vi "Key_Display.vi"(0 "Data In":T6 caption="单捞磐 涝仿", 2 "Display State In":T4 caption="叼胶敲饭捞 惑怕 涝仿", 3 "Container State":T5 caption="牧抛捞呈 惑怕") -> (6 "Data Out":T6 caption="单捞磐 免仿", 7 "Display State Out":T4 caption="叼胶敲饭捞 惑怕 免仿", 8 "Action":T3 caption="累诀")   [LabVIEW 2012, in "Key_Xcontrol.xctl"]
uses:
  Key_Xcontrol.xctl
  Key_Data.ctl
  <vilib>/_xctls/Container State.ctl
  Key_State.ctl
  <vilib>/_xctls/Action.ctl
  <vilib>/_xctls/XControlSupport.lvlib
panel:
  in  "牧飘费侩":T1
  in  "牢叼霸捞磐侩":T2
  out "DISPLAY":T7
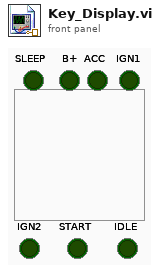
[diagram p1: front panel]
types:
  T1 = cluster{"SLEEP 2":bool, "B+ 2":bool, "ACC 2":bool, "IGN1 2":bool, "IGN2 2":bool, "START 2":bool, "IDLE 2":bool}
  T2 = cluster{"SLEEP":bool, "B+":bool, "ACC":bool, "IGN1":bool, "IGN2":bool, "START":bool, "IDLE":bool}
  T3 = typedef "XControlSupport.lvlib/Action.ctl" = cluster{"Data Changed?":bool, "State Changed?":bool, "Action Name":string}
  T4 = typedef "Key_Xcontrol.xctl/Key_State.ctl" = cluster{"Numeric":u8}
  T5 = typedef "XControlSupport.lvlib/Container State.ctl" = cluster{"Indicator?":bool, "Run Mode?":bool, " Refnum":refnum<vi>}
  T6 = typedef "Key_Xcontrol.xctl/Key_Data.ctl" = u8
  T7 = cluster{"Key In":bool, "acc":bool, "ign":bool, "start":bool}
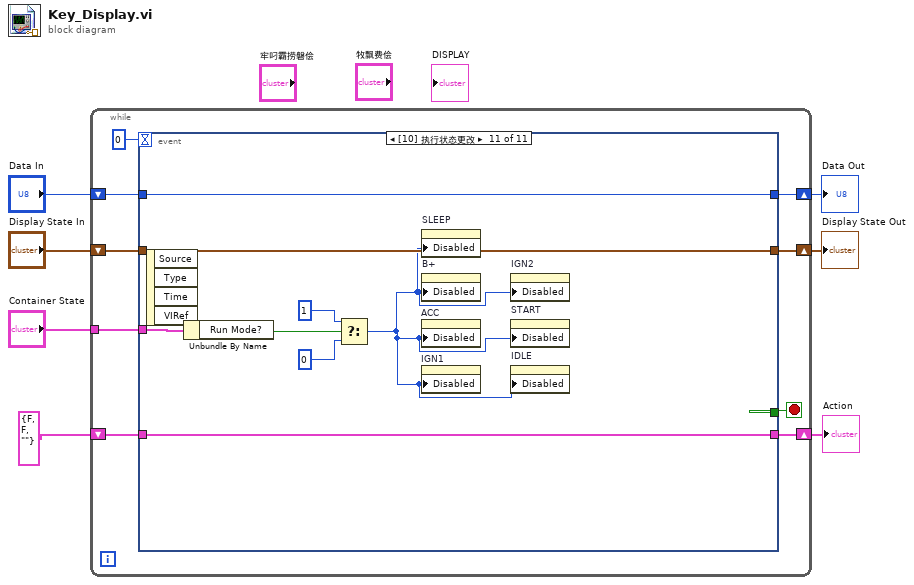
[diagram p0: block diagram]
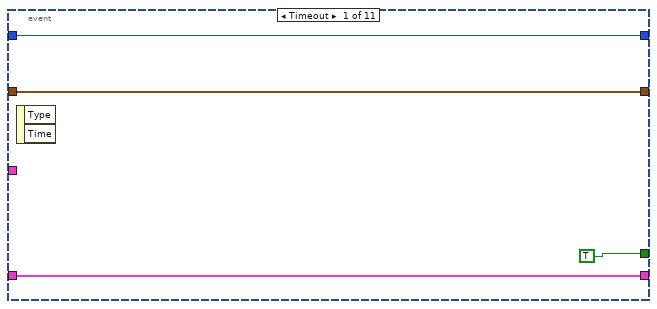
[diagram p2: hidden frame]
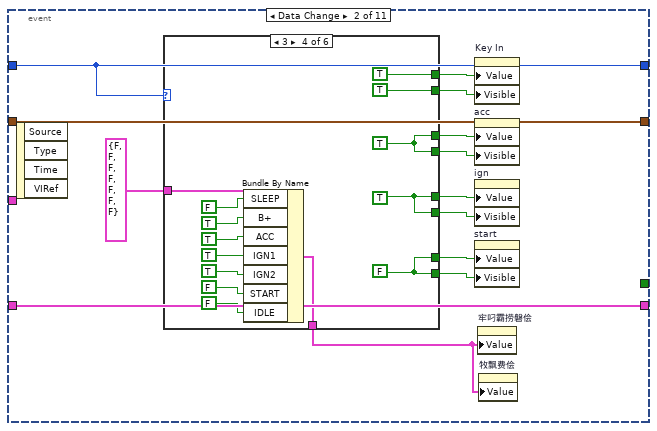
[diagram p3: hidden frame]
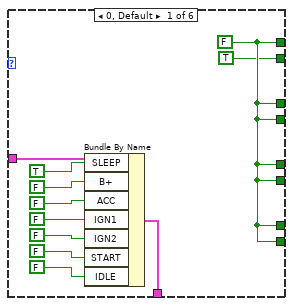
[diagram p4: hidden frame]
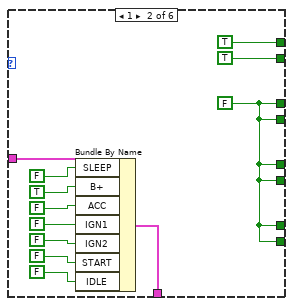
[diagram p5: hidden frame]
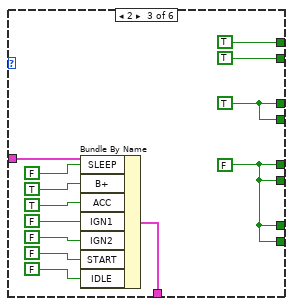
[diagram p6: hidden frame]
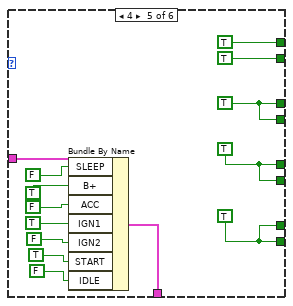
[diagram p7: hidden frame]
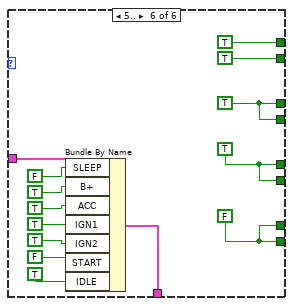
[diagram p8: hidden frame]
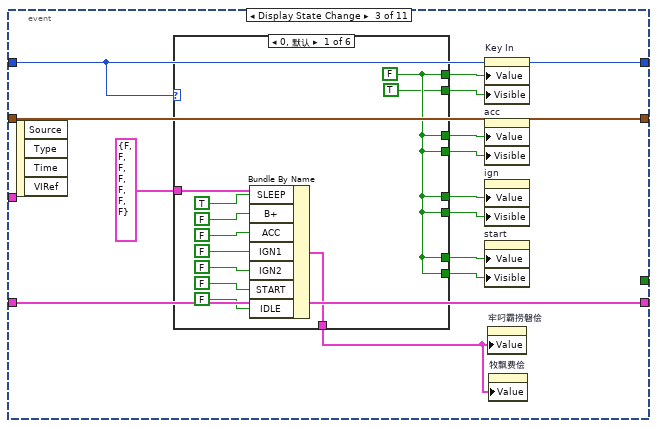
[diagram p9: hidden frame]
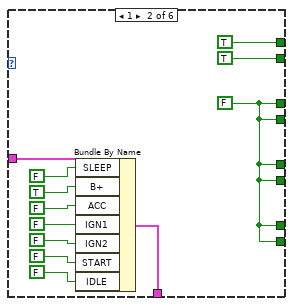
[diagram p10: hidden frame]
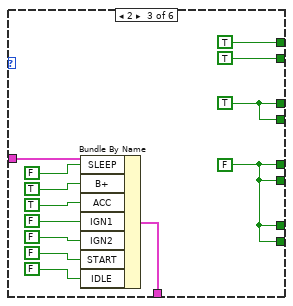
[diagram p11: hidden frame]
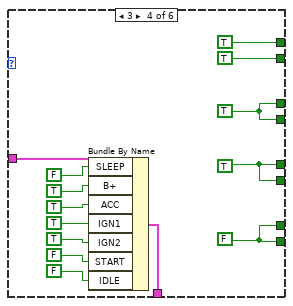
[diagram p12: hidden frame]
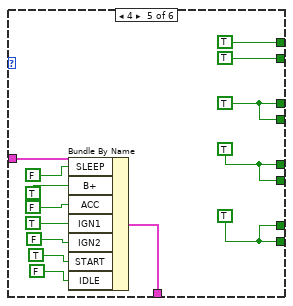
[diagram p13: hidden frame]
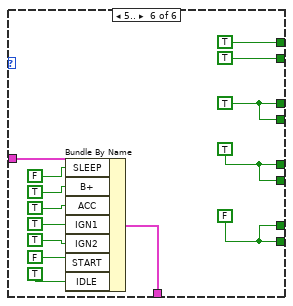
[diagram p14: hidden frame]
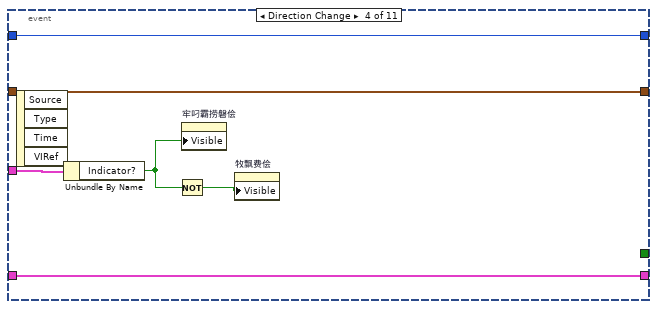
[diagram p15: hidden frame]
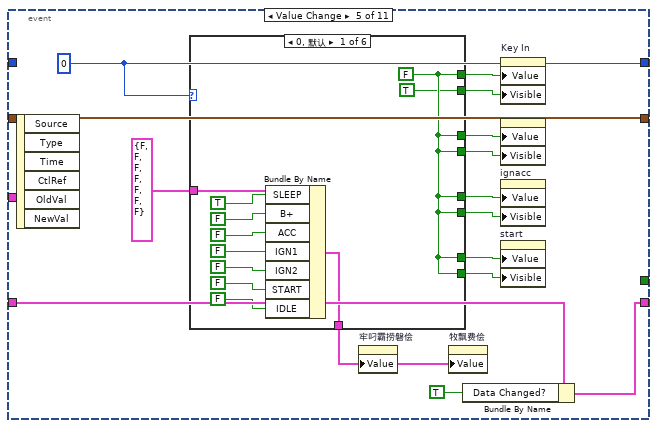
[diagram p16: hidden frame]
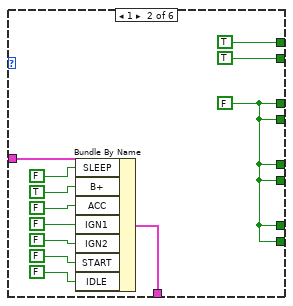
[diagram p17: hidden frame]
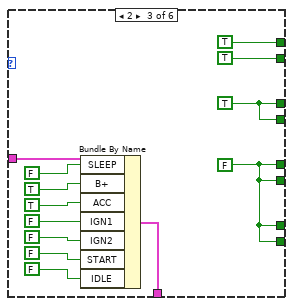
[diagram p18: hidden frame]
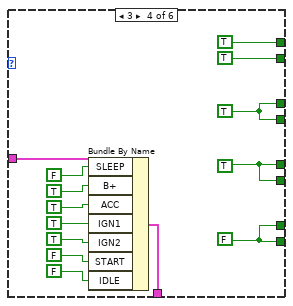
[diagram p19: hidden frame]
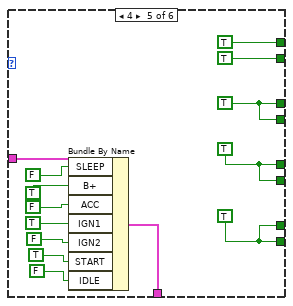
[diagram p20: hidden frame]
diagram:
  n1 = while {
    shift-right: [w15] -> w4
    shift-left: "Display State In" -> [w16]
    tunnel: "Container State" -> [w12]
    shift-right: [w10] -> w7
    shift-left: "Data In" -> [w11]
    shift-right: [w8] -> w2
    shift-left: T3 {"Data Changed?"=FALSE, "State Changed?"=FALSE, "Action Name"=""} ("Action") -> [w9]
    stop <- w14 stop-if-true
    n2 = event shown="[10] 执行状态更改" {
      selector: _ -> [_ _ _ _ _ _ _ _ _ _ _]
      dyn-events: _ -> [_ _ _ _ _ _ _ _ _ _ _]
      timeout: 0 -> [_ _ _ _ _ _ _ _ _ _ _]
      tunnel: w16 -> [w18 w33 w124 w207 w209 w316 w409 w502 w595 w688 w773]
      tunnel: [w18 w33 w124 w207 w209 w316 w409 w502 w595 w688 w773] -> w15
      tunnel: [TRUE _ _ _ _ _ _ _ _ _ _] -> w14
      tunnel: w12 -> [_ _ _ w208 _ _ _ _ _ _ w774]
      tunnel: w11 -> [w17 w31 w112 w206 _ _ _ _ _ _ w772]
      tunnel: [w17 w31 w112 w206 w210 w302 w395 w488 w581 w674 w772] -> w10
      tunnel: [w19 w32 w123 w205 w223 w313 w406 w499 w592 w685 w771] -> w8
      tunnel: w9 -> [w19 w32 w123 w205 w221 w314 w407 w500 w593 w686 w771]
      event Timeout {
        n3 = event-data() -> ()  [unwired: 1 in, 2 out]
      }
      event Data Change {
        n4 = event-data() -> ()  [unwired: 1 in, 4 out]
        n5 = case shown="3" w31 {
          tunnel: [w44 TRUE ("Key In") TRUE ("Key In") TRUE ("Key In") TRUE ("Key In") TRUE ("Key In")] -> w30
          tunnel: [TRUE ("Key In") TRUE ("Key In") TRUE ("Key In") TRUE ("Key In") TRUE ("Key In") TRUE ("Key In")] -> w29
          tunnel: [w44 w54 w67 w81 w95 w109] -> w28
          tunnel: [w44 w54 w67 w81 w95 w109] -> w27
          tunnel: [w44 w54 w66 w80 w94 w108] -> w26
          tunnel: [w44 w54 w66 w79 w93 w107] -> w25
          tunnel: [w44 w54 w66 w79 w93 w107] -> w24
          tunnel: [w44 w54 w66 w80 w94 w108] -> w23
          tunnel: T2 {"SLEEP"=FALSE, "B+"=FALSE, "ACC"=FALSE, "IGN1"=FALSE, "IGN2"=FALSE, "START"=FALSE, "IDLE"=FALSE} ("牢叼霸捞磐侩") -> [w34 w46 w58 w78 w85 w99]
          tunnel: [w35 w45 w57 w70 w84 w98] -> w21
          frame 0, Default {
            w44 = FALSE ("Key In")
            n6 = Bundle By Name(cluster=w34, "SLEEP"=TRUE, "B+"=FALSE ("SLEEP"), "ACC"=FALSE ("SLEEP"), "IGN1"=FALSE ("SLEEP"), "IGN2"=FALSE ("SLEEP"), "START"=FALSE ("SLEEP"), "IDLE"=FALSE ("SLEEP")) -> (w35:T2)
          }
          frame 1 {
            w54 = FALSE ("Key In")
            n7 = Bundle By Name(cluster=w46, "SLEEP"=FALSE, "B+"=TRUE ("SLEEP"), "ACC"=FALSE ("SLEEP"), "IGN1"=FALSE ("SLEEP"), "IGN2"=FALSE ("SLEEP"), "START"=FALSE ("SLEEP"), "IDLE"=FALSE ("SLEEP")) -> (w45:T2)
          }
          frame 2 {
            w66 = FALSE ("Key In")
            w67 = TRUE ("Key In")
            n8 = Bundle By Name(cluster=w58, "SLEEP"=FALSE, "B+"=TRUE ("SLEEP"), "ACC"=TRUE ("SLEEP"), "IGN1"=FALSE ("SLEEP"), "IGN2"=FALSE ("SLEEP"), "START"=FALSE ("SLEEP"), "IDLE"=FALSE ("SLEEP")) -> (w57:T2)
          }
          frame 3 {
            w79 = FALSE ("Key In")
            w80 = TRUE ("Key In")
            w81 = TRUE ("Key In")
            n9 = Bundle By Name(cluster=w78, "SLEEP"=FALSE, "B+"=TRUE ("SLEEP"), "ACC"=TRUE ("SLEEP"), "IGN1"=TRUE ("SLEEP"), "IGN2"=TRUE ("SLEEP"), "START"=FALSE ("SLEEP"), "IDLE"=FALSE ("SLEEP")) -> (w70:T2)
          }
          frame 4 {
            w93 = TRUE ("Key In")
            w94 = TRUE ("Key In")
            w95 = TRUE ("Key In")
            n10 = Bundle By Name(cluster=w85, "SLEEP"=FALSE, "B+"=TRUE ("SLEEP"), "ACC"=FALSE ("SLEEP"), "IGN1"=TRUE ("SLEEP"), "IGN2"=FALSE ("SLEEP"), "START"=TRUE ("SLEEP"), "IDLE"=FALSE ("SLEEP")) -> (w84:T2)
          }
          frame 5.. {
            w107 = FALSE ("Key In")
            w108 = TRUE ("Key In")
            w109 = TRUE ("Key In")
            n11 = Bundle By Name(cluster=w99, "SLEEP"=FALSE, "B+"=TRUE ("SLEEP"), "ACC"=TRUE ("SLEEP"), "IGN1"=TRUE ("SLEEP"), "IGN2"=TRUE ("SLEEP"), "START"=FALSE ("SLEEP"), "IDLE"=TRUE ("SLEEP")) -> (w98:T2)
          }
        }
        n12 = property on="Key In" class="Bool (严格)"("Value"=w30, "Visible"=w29) -> ()  [unwired: 2 in, 2 out]
        n13 = property on="acc" class="Bool (严格)"("Value"=w27, "Visible"=w28) -> ()  [unwired: 2 in, 2 out]
        n14 = property on="ign" class="Bool (严格)"("Value"=w23, "Visible"=w26) -> ()  [unwired: 2 in, 2 out]
        n15 = property on="start" class="Bool (严格)"("Value"=w24, "Visible"=w25) -> ()  [unwired: 2 in, 2 out]
        n16 = property on="牢叼霸捞磐侩" class="Clust (严格)"("Value"=w21) -> ()  [unwired: 2 in, 2 out]
        n17 = property on="牧飘费侩" class="Clust (严格)"("Value"=w21) -> ()  [unwired: 2 in, 2 out]
      }
      event Display State Change {
        n18 = event-data() -> ()  [unwired: 1 in, 4 out]
        n19 = case shown="0, 默认" w112 {
          tunnel: [w135 TRUE ("Key In") TRUE ("Key In") TRUE ("Key In") TRUE ("Key In") TRUE ("Key In")] -> w122
          tunnel: [TRUE ("Key In") TRUE ("Key In") TRUE ("Key In") TRUE ("Key In") TRUE ("Key In") TRUE ("Key In")] -> w121
          tunnel: [w135 w145 w158 w172 w186 w200] -> w120
          tunnel: [w135 w145 w158 w172 w186 w200] -> w119
          tunnel: [w135 w145 w157 w171 w185 w199] -> w118
          tunnel: [w135 w145 w157 w170 w184 w198] -> w117
          tunnel: [w135 w145 w157 w170 w184 w198] -> w116
          tunnel: [w135 w145 w157 w171 w185 w199] -> w115
          tunnel: T2 {"SLEEP"=FALSE, "B+"=FALSE, "ACC"=FALSE, "IGN1"=FALSE, "IGN2"=FALSE, "START"=FALSE, "IDLE"=FALSE} ("牢叼霸捞磐侩") -> [w125 w137 w149 w169 w176 w190]
          tunnel: [w126 w136 w148 w161 w175 w189] -> w113
          frame 0, Default {
            w135 = FALSE ("Key In")
            n20 = Bundle By Name(cluster=w125, "SLEEP"=TRUE, "B+"=FALSE ("SLEEP"), "ACC"=FALSE ("SLEEP"), "IGN1"=FALSE ("SLEEP"), "IGN2"=FALSE ("SLEEP"), "START"=FALSE ("SLEEP"), "IDLE"=FALSE ("SLEEP")) -> (w126:T2)
          }
          frame 1 {
            w145 = FALSE ("Key In")
            n21 = Bundle By Name(cluster=w137, "SLEEP"=FALSE, "B+"=TRUE ("SLEEP"), "ACC"=FALSE ("SLEEP"), "IGN1"=FALSE ("SLEEP"), "IGN2"=FALSE ("SLEEP"), "START"=FALSE ("SLEEP"), "IDLE"=FALSE ("SLEEP")) -> (w136:T2)
          }
          frame 2 {
            w157 = FALSE ("Key In")
            w158 = TRUE ("Key In")
            n22 = Bundle By Name(cluster=w149, "SLEEP"=FALSE, "B+"=TRUE ("SLEEP"), "ACC"=TRUE ("SLEEP"), "IGN1"=FALSE ("SLEEP"), "IGN2"=FALSE ("SLEEP"), "START"=FALSE ("SLEEP"), "IDLE"=FALSE ("SLEEP")) -> (w148:T2)
          }
          frame 3 {
            w170 = FALSE ("Key In")
            w171 = TRUE ("Key In")
            w172 = TRUE ("Key In")
            n23 = Bundle By Name(cluster=w169, "SLEEP"=FALSE, "B+"=TRUE ("SLEEP"), "ACC"=TRUE ("SLEEP"), "IGN1"=TRUE ("SLEEP"), "IGN2"=TRUE ("SLEEP"), "START"=FALSE ("SLEEP"), "IDLE"=FALSE ("SLEEP")) -> (w161:T2)
          }
          frame 4 {
            w184 = TRUE ("Key In")
            w185 = TRUE ("Key In")
            w186 = TRUE ("Key In")
            n24 = Bundle By Name(cluster=w176, "SLEEP"=FALSE, "B+"=TRUE ("SLEEP"), "ACC"=FALSE ("SLEEP"), "IGN1"=TRUE ("SLEEP"), "IGN2"=FALSE ("SLEEP"), "START"=TRUE ("SLEEP"), "IDLE"=FALSE ("SLEEP")) -> (w175:T2)
          }
          frame 5.. {
            w198 = FALSE ("Key In")
            w199 = TRUE ("Key In")
            w200 = TRUE ("Key In")
            n25 = Bundle By Name(cluster=w190, "SLEEP"=FALSE, "B+"=TRUE ("SLEEP"), "ACC"=TRUE ("SLEEP"), "IGN1"=TRUE ("SLEEP"), "IGN2"=TRUE ("SLEEP"), "START"=FALSE ("SLEEP"), "IDLE"=TRUE ("SLEEP")) -> (w189:T2)
          }
        }
        n26 = property on="Key In" class="Bool (严格)"("Value"=w122, "Visible"=w121) -> ()  [unwired: 2 in, 2 out]
        n27 = property on="acc" class="Bool (严格)"("Value"=w119, "Visible"=w120) -> ()  [unwired: 2 in, 2 out]
        n28 = property on="ign" class="Bool (严格)"("Value"=w115, "Visible"=w118) -> ()  [unwired: 2 in, 2 out]
        n29 = property on="start" class="Bool (严格)"("Value"=w116, "Visible"=w117) -> ()  [unwired: 2 in, 2 out]
        n30 = property on="牢叼霸捞磐侩" class="Clust (严格)"("Value"=w113) -> ()  [unwired: 2 in, 2 out]
        n31 = property on="牧飘费侩" class="Clust (严格)"("Value"=w113) -> ()  [unwired: 2 in, 2 out]
      }
      event Direction Change {
        n32 = event-data() -> ()  [unwired: 1 in, 4 out]
        n33 = Unbundle By Name(w208) -> ("Indicator?"=w204:bool)
        n34 = Not(x=w204) -> (.not. x?=w203:bool)
        n35 = property on="牢叼霸捞磐侩" class="Clust (严格)"("Visible"=w204) -> ()  [unwired: 2 in, 2 out]
        n36 = property on="牧飘费侩" class="Clust (严格)"("Visible"=w203) -> ()  [unwired: 2 in, 2 out]
      }
      event "牢叼霸捞磐侩.SLEEP", "牧飘费侩.SLEEP 2": Value Change {
        w210 = T6 0 ("Data In")
        n37 = event-data() -> ()  [unwired: 1 in, 6 out]
        n38 = case shown="0, 默认" w210 {
          tunnel: [w234 TRUE ("Key In") TRUE ("Key In") TRUE ("Key In") TRUE ("Key In") TRUE ("Key In")] -> w220
          tunnel: [TRUE ("Key In") TRUE ("Key In") TRUE ("Key In") TRUE ("Key In") TRUE ("Key In") TRUE ("Key In")] -> w219
          tunnel: [w234 w244 w257 w271 w285 w299] -> w218
          tunnel: [w234 w244 w257 w271 w285 w299] -> w217
          tunnel: [w234 w244 w256 w270 w284 w298] -> w216
          tunnel: [w234 w244 w256 w269 w283 w297] -> w215
          tunnel: [w234 w244 w256 w269 w283 w297] -> w214
          tunnel: [w234 w244 w256 w270 w284 w298] -> w213
          tunnel: T2 {"SLEEP"=FALSE, "B+"=FALSE, "ACC"=FALSE, "IGN1"=FALSE, "IGN2"=FALSE, "START"=FALSE, "IDLE"=FALSE} ("牢叼霸捞磐侩") -> [w224 w236 w248 w268 w275 w289]
          tunnel: [w225 w235 w247 w260 w274 w288] -> w211
          frame 0, Default {
            w234 = FALSE ("Key In")
            n39 = Bundle By Name(cluster=w224, "SLEEP"=TRUE, "B+"=FALSE ("SLEEP"), "ACC"=FALSE ("SLEEP"), "IGN1"=FALSE ("SLEEP"), "IGN2"=FALSE ("SLEEP"), "START"=FALSE ("SLEEP"), "IDLE"=FALSE ("SLEEP")) -> (w225:T2)
          }
          frame 1 {
            w244 = FALSE ("Key In")
            n40 = Bundle By Name(cluster=w236, "SLEEP"=FALSE, "B+"=TRUE ("SLEEP"), "ACC"=FALSE ("SLEEP"), "IGN1"=FALSE ("SLEEP"), "IGN2"=FALSE ("SLEEP"), "START"=FALSE ("SLEEP"), "IDLE"=FALSE ("SLEEP")) -> (w235:T2)
          }
          frame 2 {
            w256 = FALSE ("Key In")
            w257 = TRUE ("Key In")
            n41 = Bundle By Name(cluster=w248, "SLEEP"=FALSE, "B+"=TRUE ("SLEEP"), "ACC"=TRUE ("SLEEP"), "IGN1"=FALSE ("SLEEP"), "IGN2"=FALSE ("SLEEP"), "START"=FALSE ("SLEEP"), "IDLE"=FALSE ("SLEEP")) -> (w247:T2)
          }
          frame 3 {
            w269 = FALSE ("Key In")
            w270 = TRUE ("Key In")
            w271 = TRUE ("Key In")
            n42 = Bundle By Name(cluster=w268, "SLEEP"=FALSE, "B+"=TRUE ("SLEEP"), "ACC"=TRUE ("SLEEP"), "IGN1"=TRUE ("SLEEP"), "IGN2"=TRUE ("SLEEP"), "START"=FALSE ("SLEEP"), "IDLE"=FALSE ("SLEEP")) -> (w260:T2)
          }
          frame 4 {
            w283 = TRUE ("Key In")
            w284 = TRUE ("Key In")
            w285 = TRUE ("Key In")
            n43 = Bundle By Name(cluster=w275, "SLEEP"=FALSE, "B+"=TRUE ("SLEEP"), "ACC"=FALSE ("SLEEP"), "IGN1"=TRUE ("SLEEP"), "IGN2"=FALSE ("SLEEP"), "START"=TRUE ("SLEEP"), "IDLE"=FALSE ("SLEEP")) -> (w274:T2)
          }
          frame 5.. {
            w297 = FALSE ("Key In")
            w298 = TRUE ("Key In")
            w299 = TRUE ("Key In")
            n44 = Bundle By Name(cluster=w289, "SLEEP"=FALSE, "B+"=TRUE ("SLEEP"), "ACC"=TRUE ("SLEEP"), "IGN1"=TRUE ("SLEEP"), "IGN2"=TRUE ("SLEEP"), "START"=FALSE ("SLEEP"), "IDLE"=TRUE ("SLEEP")) -> (w288:T2)
          }
        }
        n45 = property on="牢叼霸捞磐侩" class="Clust (严格)"("Value"=w211) -> ()  [unwired: 2 in, 2 out]
        n46 = property on="牧飘费侩" class="Clust (严格)"("Value"=w211) -> ()  [unwired: 2 in, 2 out]
        n47 = Bundle By Name(cluster=w221, "Data Changed?"=TRUE) -> (w223:T3)
        n48 = property on="Key In" class="Bool (严格)"("Value"=w220, "Visible"=w219) -> ()  [unwired: 2 in, 2 out]
        n49 = property on="acc" class="Bool (严格)"("Value"=w217, "Visible"=w218) -> ()  [unwired: 2 in, 2 out]
        n50 = property on="ign" class="Bool (严格)"("Value"=w213, "Visible"=w216) -> ()  [unwired: 2 in, 2 out]
        n51 = property on="start" class="Bool (严格)"("Value"=w214, "Visible"=w215) -> ()  [unwired: 2 in, 2 out]
      }
      event "牢叼霸捞磐侩.B+", "牧飘费侩.B+ 2": Value Change {
        w302 = T6 1 ("Data In")
        n52 = event-data() -> ()  [unwired: 1 in, 6 out]
        n53 = case shown="0, 默认" w302 {
          tunnel: [w327 TRUE ("Key In") TRUE ("Key In") TRUE ("Key In") TRUE ("Key In") TRUE ("Key In")] -> w312
          tunnel: [TRUE ("Key In") TRUE ("Key In") TRUE ("Key In") TRUE ("Key In") TRUE ("Key In") TRUE ("Key In")] -> w311
          tunnel: [w327 w337 w350 w364 w378 w392] -> w310
          tunnel: [w327 w337 w350 w364 w378 w392] -> w309
          tunnel: [w327 w337 w349 w363 w377 w391] -> w308
          tunnel: [w327 w337 w349 w362 w376 w390] -> w307
          tunnel: [w327 w337 w349 w362 w376 w390] -> w306
          tunnel: [w327 w337 w349 w363 w377 w391] -> w305
          tunnel: T2 {"SLEEP"=FALSE, "B+"=FALSE, "ACC"=FALSE, "IGN1"=FALSE, "IGN2"=FALSE, "START"=FALSE, "IDLE"=FALSE} ("牢叼霸捞磐侩") -> [w317 w329 w341 w361 w368 w382]
          tunnel: [w318 w328 w340 w353 w367 w381] -> w303
          frame 0, Default {
            w327 = FALSE ("Key In")
            n54 = Bundle By Name(cluster=w317, "SLEEP"=TRUE, "B+"=FALSE ("SLEEP"), "ACC"=FALSE ("SLEEP"), "IGN1"=FALSE ("SLEEP"), "IGN2"=FALSE ("SLEEP"), "START"=FALSE ("SLEEP"), "IDLE"=FALSE ("SLEEP")) -> (w318:T2)
          }
          frame 1 {
            w337 = FALSE ("Key In")
            n55 = Bundle By Name(cluster=w329, "SLEEP"=FALSE, "B+"=TRUE ("SLEEP"), "ACC"=FALSE ("SLEEP"), "IGN1"=FALSE ("SLEEP"), "IGN2"=FALSE ("SLEEP"), "START"=FALSE ("SLEEP"), "IDLE"=FALSE ("SLEEP")) -> (w328:T2)
          }
          frame 2 {
            w349 = FALSE ("Key In")
            w350 = TRUE ("Key In")
            n56 = Bundle By Name(cluster=w341, "SLEEP"=FALSE, "B+"=TRUE ("SLEEP"), "ACC"=TRUE ("SLEEP"), "IGN1"=FALSE ("SLEEP"), "IGN2"=FALSE ("SLEEP"), "START"=FALSE ("SLEEP"), "IDLE"=FALSE ("SLEEP")) -> (w340:T2)
          }
          frame 3 {
            w362 = FALSE ("Key In")
            w363 = TRUE ("Key In")
            w364 = TRUE ("Key In")
            n57 = Bundle By Name(cluster=w361, "SLEEP"=FALSE, "B+"=TRUE ("SLEEP"), "ACC"=TRUE ("SLEEP"), "IGN1"=TRUE ("SLEEP"), "IGN2"=TRUE ("SLEEP"), "START"=FALSE ("SLEEP"), "IDLE"=FALSE ("SLEEP")) -> (w353:T2)
          }
          frame 4 {
            w376 = TRUE ("Key In")
            w377 = TRUE ("Key In")
            w378 = TRUE ("Key In")
            n58 = Bundle By Name(cluster=w368, "SLEEP"=FALSE, "B+"=TRUE ("SLEEP"), "ACC"=FALSE ("SLEEP"), "IGN1"=TRUE ("SLEEP"), "IGN2"=FALSE ("SLEEP"), "START"=TRUE ("SLEEP"), "IDLE"=FALSE ("SLEEP")) -> (w367:T2)
          }
          frame 5.. {
            w390 = FALSE ("Key In")
            w391 = TRUE ("Key In")
            w392 = TRUE ("Key In")
            n59 = Bundle By Name(cluster=w382, "SLEEP"=FALSE, "B+"=TRUE ("SLEEP"), "ACC"=TRUE ("SLEEP"), "IGN1"=TRUE ("SLEEP"), "IGN2"=TRUE ("SLEEP"), "START"=FALSE ("SLEEP"), "IDLE"=TRUE ("SLEEP")) -> (w381:T2)
          }
        }
        n60 = property on="牢叼霸捞磐侩" class="Clust (严格)"("Value"=w303) -> ()  [unwired: 2 in, 2 out]
        n61 = Bundle By Name(cluster=w314, "Data Changed?"=TRUE) -> (w313:T3)
        n62 = property on="牧飘费侩" class="Clust (严格)"("Value"=w303) -> ()  [unwired: 2 in, 2 out]
        n63 = property on="Key In" class="Bool (严格)"("Value"=w312, "Visible"=w311) -> ()  [unwired: 2 in, 2 out]
        n64 = property on="acc" class="Bool (严格)"("Value"=w309, "Visible"=w310) -> ()  [unwired: 2 in, 2 out]
        n65 = property on="ign" class="Bool (严格)"("Value"=w305, "Visible"=w308) -> ()  [unwired: 2 in, 2 out]
        n66 = property on="start" class="Bool (严格)"("Value"=w306, "Visible"=w307) -> ()  [unwired: 2 in, 2 out]
      }
      event "牢叼霸捞磐侩.ACC", "牧飘费侩.ACC 2": Value Change {
        w395 = T6 2 ("Data In")
        n67 = event-data() -> ()  [unwired: 1 in, 6 out]
        n68 = case shown="0, 默认" w395 {
          tunnel: [w420 TRUE ("Key In") TRUE ("Key In") TRUE ("Key In") TRUE ("Key In") TRUE ("Key In")] -> w405
          tunnel: [TRUE ("Key In") TRUE ("Key In") TRUE ("Key In") TRUE ("Key In") TRUE ("Key In") TRUE ("Key In")] -> w404
          tunnel: [w420 w430 w443 w457 w471 w485] -> w403
          tunnel: [w420 w430 w443 w457 w471 w485] -> w402
          tunnel: [w420 w430 w442 w456 w470 w484] -> w401
          tunnel: [w420 w430 w442 w455 w469 w483] -> w400
          tunnel: [w420 w430 w442 w455 w469 w483] -> w399
          tunnel: [w420 w430 w442 w456 w470 w484] -> w398
          tunnel: T2 {"SLEEP"=FALSE, "B+"=FALSE, "ACC"=FALSE, "IGN1"=FALSE, "IGN2"=FALSE, "START"=FALSE, "IDLE"=FALSE} ("牢叼霸捞磐侩") -> [w410 w422 w434 w454 w461 w475]
          tunnel: [w411 w421 w433 w446 w460 w474] -> w396
          frame 0, Default {
            w420 = FALSE ("Key In")
            n69 = Bundle By Name(cluster=w410, "SLEEP"=TRUE, "B+"=FALSE ("SLEEP"), "ACC"=FALSE ("SLEEP"), "IGN1"=FALSE ("SLEEP"), "IGN2"=FALSE ("SLEEP"), "START"=FALSE ("SLEEP"), "IDLE"=FALSE ("SLEEP")) -> (w411:T2)
          }
          frame 1 {
            w430 = FALSE ("Key In")
            n70 = Bundle By Name(cluster=w422, "SLEEP"=FALSE, "B+"=TRUE ("SLEEP"), "ACC"=FALSE ("SLEEP"), "IGN1"=FALSE ("SLEEP"), "IGN2"=FALSE ("SLEEP"), "START"=FALSE ("SLEEP"), "IDLE"=FALSE ("SLEEP")) -> (w421:T2)
          }
          frame 2 {
            w442 = FALSE ("Key In")
            w443 = TRUE ("Key In")
            n71 = Bundle By Name(cluster=w434, "SLEEP"=FALSE, "B+"=TRUE ("SLEEP"), "ACC"=TRUE ("SLEEP"), "IGN1"=FALSE ("SLEEP"), "IGN2"=FALSE ("SLEEP"), "START"=FALSE ("SLEEP"), "IDLE"=FALSE ("SLEEP")) -> (w433:T2)
          }
          frame 3 {
            w455 = FALSE ("Key In")
            w456 = TRUE ("Key In")
            w457 = TRUE ("Key In")
            n72 = Bundle By Name(cluster=w454, "SLEEP"=FALSE, "B+"=TRUE ("SLEEP"), "ACC"=TRUE ("SLEEP"), "IGN1"=TRUE ("SLEEP"), "IGN2"=TRUE ("SLEEP"), "START"=FALSE ("SLEEP"), "IDLE"=FALSE ("SLEEP")) -> (w446:T2)
          }
          frame 4 {
            w469 = TRUE ("Key In")
            w470 = TRUE ("Key In")
            w471 = TRUE ("Key In")
            n73 = Bundle By Name(cluster=w461, "SLEEP"=FALSE, "B+"=TRUE ("SLEEP"), "ACC"=FALSE ("SLEEP"), "IGN1"=TRUE ("SLEEP"), "IGN2"=FALSE ("SLEEP"), "START"=TRUE ("SLEEP"), "IDLE"=FALSE ("SLEEP")) -> (w460:T2)
          }
          frame 5.. {
            w483 = FALSE ("Key In")
            w484 = TRUE ("Key In")
            w485 = TRUE ("Key In")
            n74 = Bundle By Name(cluster=w475, "SLEEP"=FALSE, "B+"=TRUE ("SLEEP"), "ACC"=TRUE ("SLEEP"), "IGN1"=TRUE ("SLEEP"), "IGN2"=TRUE ("SLEEP"), "START"=FALSE ("SLEEP"), "IDLE"=TRUE ("SLEEP")) -> (w474:T2)
          }
        }
        n75 = property on="牢叼霸捞磐侩" class="Clust (严格)"("Value"=w396) -> ()  [unwired: 2 in, 2 out]
        n76 = Bundle By Name(cluster=w407, "Data Changed?"=TRUE) -> (w406:T3)
        n77 = property on="牧飘费侩" class="Clust (严格)"("Value"=w396) -> ()  [unwired: 2 in, 2 out]
        n78 = property on="Key In" class="Bool (严格)"("Value"=w405, "Visible"=w404) -> ()  [unwired: 2 in, 2 out]
        n79 = property on="acc" class="Bool (严格)"("Value"=w402, "Visible"=w403) -> ()  [unwired: 2 in, 2 out]
        n80 = property on="ign" class="Bool (严格)"("Value"=w398, "Visible"=w401) -> ()  [unwired: 2 in, 2 out]
        n81 = property on="start" class="Bool (严格)"("Value"=w399, "Visible"=w400) -> ()  [unwired: 2 in, 2 out]
      }
      event "牢叼霸捞磐侩.IGN1", "牢叼霸捞磐侩.IGN2", "牧飘费侩.IGN1 2", "牧飘费侩.IGN2 2": Value Change {
        w488 = T6 3 ("Data In")
        n82 = event-data() -> ()  [unwired: 1 in, 6 out]
        n83 = case shown="0, 默认" w488 {
          tunnel: [w513 TRUE ("Key In") TRUE ("Key In") TRUE ("Key In") TRUE ("Key In") TRUE ("Key In")] -> w498
          tunnel: [TRUE ("Key In") TRUE ("Key In") TRUE ("Key In") TRUE ("Key In") TRUE ("Key In") TRUE ("Key In")] -> w497
          tunnel: [w513 w523 w536 w550 w564 w578] -> w496
          tunnel: [w513 w523 w536 w550 w564 w578] -> w495
          tunnel: [w513 w523 w535 w549 w563 w577] -> w494
          tunnel: [w513 w523 w535 w548 w562 w576] -> w493
          tunnel: [w513 w523 w535 w548 w562 w576] -> w492
          tunnel: [w513 w523 w535 w549 w563 w577] -> w491
          tunnel: T2 {"SLEEP"=FALSE, "B+"=FALSE, "ACC"=FALSE, "IGN1"=FALSE, "IGN2"=FALSE, "START"=FALSE, "IDLE"=FALSE} ("牢叼霸捞磐侩") -> [w503 w515 w527 w547 w554 w568]
          tunnel: [w504 w514 w526 w539 w553 w567] -> w489
          frame 0, Default {
            w513 = FALSE ("Key In")
            n84 = Bundle By Name(cluster=w503, "SLEEP"=TRUE, "B+"=FALSE ("SLEEP"), "ACC"=FALSE ("SLEEP"), "IGN1"=FALSE ("SLEEP"), "IGN2"=FALSE ("SLEEP"), "START"=FALSE ("SLEEP"), "IDLE"=FALSE ("SLEEP")) -> (w504:T2)
          }
          frame 1 {
            w523 = FALSE ("Key In")
            n85 = Bundle By Name(cluster=w515, "SLEEP"=FALSE, "B+"=TRUE ("SLEEP"), "ACC"=FALSE ("SLEEP"), "IGN1"=FALSE ("SLEEP"), "IGN2"=FALSE ("SLEEP"), "START"=FALSE ("SLEEP"), "IDLE"=FALSE ("SLEEP")) -> (w514:T2)
          }
          frame 2 {
            w535 = FALSE ("Key In")
            w536 = TRUE ("Key In")
            n86 = Bundle By Name(cluster=w527, "SLEEP"=FALSE, "B+"=TRUE ("SLEEP"), "ACC"=TRUE ("SLEEP"), "IGN1"=FALSE ("SLEEP"), "IGN2"=FALSE ("SLEEP"), "START"=FALSE ("SLEEP"), "IDLE"=FALSE ("SLEEP")) -> (w526:T2)
          }
          frame 3 {
            w548 = FALSE ("Key In")
            w549 = TRUE ("Key In")
            w550 = TRUE ("Key In")
            n87 = Bundle By Name(cluster=w547, "SLEEP"=FALSE, "B+"=TRUE ("SLEEP"), "ACC"=TRUE ("SLEEP"), "IGN1"=TRUE ("SLEEP"), "IGN2"=TRUE ("SLEEP"), "START"=FALSE ("SLEEP"), "IDLE"=FALSE ("SLEEP")) -> (w539:T2)
          }
          frame 4 {
            w562 = TRUE ("Key In")
            w563 = TRUE ("Key In")
            w564 = TRUE ("Key In")
            n88 = Bundle By Name(cluster=w554, "SLEEP"=FALSE, "B+"=TRUE ("SLEEP"), "ACC"=FALSE ("SLEEP"), "IGN1"=TRUE ("SLEEP"), "IGN2"=FALSE ("SLEEP"), "START"=TRUE ("SLEEP"), "IDLE"=FALSE ("SLEEP")) -> (w553:T2)
          }
          frame 5.. {
            w576 = FALSE ("Key In")
            w577 = TRUE ("Key In")
            w578 = TRUE ("Key In")
            n89 = Bundle By Name(cluster=w568, "SLEEP"=FALSE, "B+"=TRUE ("SLEEP"), "ACC"=TRUE ("SLEEP"), "IGN1"=TRUE ("SLEEP"), "IGN2"=TRUE ("SLEEP"), "START"=FALSE ("SLEEP"), "IDLE"=TRUE ("SLEEP")) -> (w567:T2)
          }
        }
        n90 = property on="牢叼霸捞磐侩" class="Clust (严格)"("Value"=w489) -> ()  [unwired: 2 in, 2 out]
        n91 = Bundle By Name(cluster=w500, "Data Changed?"=TRUE) -> (w499:T3)
        n92 = property on="牧飘费侩" class="Clust (严格)"("Value"=w489) -> ()  [unwired: 2 in, 2 out]
        n93 = property on="Key In" class="Bool (严格)"("Value"=w498, "Visible"=w497) -> ()  [unwired: 2 in, 2 out]
        n94 = property on="acc" class="Bool (严格)"("Value"=w495, "Visible"=w496) -> ()  [unwired: 2 in, 2 out]
        n95 = property on="ign" class="Bool (严格)"("Value"=w491, "Visible"=w494) -> ()  [unwired: 2 in, 2 out]
        n96 = property on="start" class="Bool (严格)"("Value"=w492, "Visible"=w493) -> ()  [unwired: 2 in, 2 out]
      }
      event "牢叼霸捞磐侩.START", "牧飘费侩.START 2": Value Change {
        w581 = T6 4 ("Data In")
        n97 = event-data() -> ()  [unwired: 1 in, 6 out]
        n98 = case shown="0, 默认" w581 {
          tunnel: [w606 TRUE ("Key In") TRUE ("Key In") TRUE ("Key In") TRUE ("Key In") TRUE ("Key In")] -> w591
          tunnel: [TRUE ("Key In") TRUE ("Key In") TRUE ("Key In") TRUE ("Key In") TRUE ("Key In") TRUE ("Key In")] -> w590
          tunnel: [w606 w616 w629 w643 w657 w671] -> w589
          tunnel: [w606 w616 w629 w643 w657 w671] -> w588
          tunnel: [w606 w616 w628 w642 w656 w670] -> w587
          tunnel: [w606 w616 w628 w641 w655 w669] -> w586
          tunnel: [w606 w616 w628 w641 w655 w669] -> w585
          tunnel: [w606 w616 w628 w642 w656 w670] -> w584
          tunnel: T2 {"SLEEP"=FALSE, "B+"=FALSE, "ACC"=FALSE, "IGN1"=FALSE, "IGN2"=FALSE, "START"=FALSE, "IDLE"=FALSE} ("牢叼霸捞磐侩") -> [w596 w608 w620 w640 w647 w661]
          tunnel: [w597 w607 w619 w632 w646 w660] -> w582
          frame 0, Default {
            w606 = FALSE ("Key In")
            n99 = Bundle By Name(cluster=w596, "SLEEP"=TRUE, "B+"=FALSE ("SLEEP"), "ACC"=FALSE ("SLEEP"), "IGN1"=FALSE ("SLEEP"), "IGN2"=FALSE ("SLEEP"), "START"=FALSE ("SLEEP"), "IDLE"=FALSE ("SLEEP")) -> (w597:T2)
          }
          frame 1 {
            w616 = FALSE ("Key In")
            n100 = Bundle By Name(cluster=w608, "SLEEP"=FALSE, "B+"=TRUE ("SLEEP"), "ACC"=FALSE ("SLEEP"), "IGN1"=FALSE ("SLEEP"), "IGN2"=FALSE ("SLEEP"), "START"=FALSE ("SLEEP"), "IDLE"=FALSE ("SLEEP")) -> (w607:T2)
          }
          frame 2 {
            w628 = FALSE ("Key In")
            w629 = TRUE ("Key In")
            n101 = Bundle By Name(cluster=w620, "SLEEP"=FALSE, "B+"=TRUE ("SLEEP"), "ACC"=TRUE ("SLEEP"), "IGN1"=FALSE ("SLEEP"), "IGN2"=FALSE ("SLEEP"), "START"=FALSE ("SLEEP"), "IDLE"=FALSE ("SLEEP")) -> (w619:T2)
          }
          frame 3 {
            w641 = FALSE ("Key In")
            w642 = TRUE ("Key In")
            w643 = TRUE ("Key In")
            n102 = Bundle By Name(cluster=w640, "SLEEP"=FALSE, "B+"=TRUE ("SLEEP"), "ACC"=TRUE ("SLEEP"), "IGN1"=TRUE ("SLEEP"), "IGN2"=TRUE ("SLEEP"), "START"=FALSE ("SLEEP"), "IDLE"=FALSE ("SLEEP")) -> (w632:T2)
          }
          frame 4 {
            w655 = TRUE ("Key In")
            w656 = TRUE ("Key In")
            w657 = TRUE ("Key In")
            n103 = Bundle By Name(cluster=w647, "SLEEP"=FALSE, "B+"=TRUE ("SLEEP"), "ACC"=FALSE ("SLEEP"), "IGN1"=TRUE ("SLEEP"), "IGN2"=FALSE ("SLEEP"), "START"=TRUE ("SLEEP"), "IDLE"=FALSE ("SLEEP")) -> (w646:T2)
          }
          frame 5.. {
            w669 = FALSE ("Key In")
            w670 = TRUE ("Key In")
            w671 = TRUE ("Key In")
            n104 = Bundle By Name(cluster=w661, "SLEEP"=FALSE, "B+"=TRUE ("SLEEP"), "ACC"=TRUE ("SLEEP"), "IGN1"=TRUE ("SLEEP"), "IGN2"=TRUE ("SLEEP"), "START"=FALSE ("SLEEP"), "IDLE"=TRUE ("SLEEP")) -> (w660:T2)
          }
        }
        n105 = property on="牢叼霸捞磐侩" class="Clust (严格)"("Value"=w582) -> ()  [unwired: 2 in, 2 out]
        n106 = Bundle By Name(cluster=w593, "Data Changed?"=TRUE) -> (w592:T3)
        n107 = property on="牧飘费侩" class="Clust (严格)"("Value"=w582) -> ()  [unwired: 2 in, 2 out]
        n108 = property on="Key In" class="Bool (严格)"("Value"=w591, "Visible"=w590) -> ()  [unwired: 2 in, 2 out]
        n109 = property on="acc" class="Bool (严格)"("Value"=w588, "Visible"=w589) -> ()  [unwired: 2 in, 2 out]
        n110 = property on="ign" class="Bool (严格)"("Value"=w584, "Visible"=w587) -> ()  [unwired: 2 in, 2 out]
        n111 = property on="start" class="Bool (严格)"("Value"=w585, "Visible"=w586) -> ()  [unwired: 2 in, 2 out]
      }
      event "牢叼霸捞磐侩.IDLE", "牧飘费侩.IDLE 2": Value Change {
        w674 = T6 5 ("Data In")
        n112 = event-data() -> ()  [unwired: 1 in, 6 out]
        n113 = case shown="0, 默认" w674 {
          tunnel: [w699 TRUE ("Key In") TRUE ("Key In") TRUE ("Key In") TRUE ("Key In") TRUE ("Key In")] -> w684
          tunnel: [TRUE ("Key In") TRUE ("Key In") TRUE ("Key In") TRUE ("Key In") TRUE ("Key In") TRUE ("Key In")] -> w683
          tunnel: [w699 w709 w722 w736 w750 w764] -> w682
          tunnel: [w699 w709 w722 w736 w750 w764] -> w681
          tunnel: [w699 w709 w721 w735 w749 w763] -> w680
          tunnel: [w699 w709 w721 w734 w748 w762] -> w679
          tunnel: [w699 w709 w721 w734 w748 w762] -> w678
          tunnel: [w699 w709 w721 w735 w749 w763] -> w677
          tunnel: T2 {"SLEEP"=FALSE, "B+"=FALSE, "ACC"=FALSE, "IGN1"=FALSE, "IGN2"=FALSE, "START"=FALSE, "IDLE"=FALSE} ("牢叼霸捞磐侩") -> [w689 w701 w713 w733 w740 w754]
          tunnel: [w690 w700 w712 w725 w739 w753] -> w675
          frame 0, Default {
            w699 = FALSE ("Key In")
            n114 = Bundle By Name(cluster=w689, "SLEEP"=TRUE, "B+"=FALSE ("SLEEP"), "ACC"=FALSE ("SLEEP"), "IGN1"=FALSE ("SLEEP"), "IGN2"=FALSE ("SLEEP"), "START"=FALSE ("SLEEP"), "IDLE"=FALSE ("SLEEP")) -> (w690:T2)
          }
          frame 1 {
            w709 = FALSE ("Key In")
            n115 = Bundle By Name(cluster=w701, "SLEEP"=FALSE, "B+"=TRUE ("SLEEP"), "ACC"=FALSE ("SLEEP"), "IGN1"=FALSE ("SLEEP"), "IGN2"=FALSE ("SLEEP"), "START"=FALSE ("SLEEP"), "IDLE"=FALSE ("SLEEP")) -> (w700:T2)
          }
          frame 2 {
            w721 = FALSE ("Key In")
            w722 = TRUE ("Key In")
            n116 = Bundle By Name(cluster=w713, "SLEEP"=FALSE, "B+"=TRUE ("SLEEP"), "ACC"=TRUE ("SLEEP"), "IGN1"=FALSE ("SLEEP"), "IGN2"=FALSE ("SLEEP"), "START"=FALSE ("SLEEP"), "IDLE"=FALSE ("SLEEP")) -> (w712:T2)
          }
          frame 3 {
            w734 = FALSE ("Key In")
            w735 = TRUE ("Key In")
            w736 = TRUE ("Key In")
            n117 = Bundle By Name(cluster=w733, "SLEEP"=FALSE, "B+"=TRUE ("SLEEP"), "ACC"=TRUE ("SLEEP"), "IGN1"=TRUE ("SLEEP"), "IGN2"=TRUE ("SLEEP"), "START"=FALSE ("SLEEP"), "IDLE"=FALSE ("SLEEP")) -> (w725:T2)
          }
          frame 4 {
            w748 = TRUE ("Key In")
            w749 = TRUE ("Key In")
            w750 = TRUE ("Key In")
            n118 = Bundle By Name(cluster=w740, "SLEEP"=FALSE, "B+"=TRUE ("SLEEP"), "ACC"=FALSE ("SLEEP"), "IGN1"=TRUE ("SLEEP"), "IGN2"=FALSE ("SLEEP"), "START"=TRUE ("SLEEP"), "IDLE"=FALSE ("SLEEP")) -> (w739:T2)
          }
          frame 5.. {
            w762 = FALSE ("Key In")
            w763 = TRUE ("Key In")
            w764 = TRUE ("Key In")
            n119 = Bundle By Name(cluster=w754, "SLEEP"=FALSE, "B+"=TRUE ("SLEEP"), "ACC"=TRUE ("SLEEP"), "IGN1"=TRUE ("SLEEP"), "IGN2"=TRUE ("SLEEP"), "START"=FALSE ("SLEEP"), "IDLE"=TRUE ("SLEEP")) -> (w753:T2)
          }
        }
        n120 = property on="牢叼霸捞磐侩" class="Clust (严格)"("Value"=w675) -> ()  [unwired: 2 in, 2 out]
        n121 = Bundle By Name(cluster=w686, "Data Changed?"=TRUE) -> (w685:T3)
        n122 = property on="牧飘费侩" class="Clust (严格)"("Value"=w675) -> ()  [unwired: 2 in, 2 out]
        n123 = property on="Key In" class="Bool (严格)"("Value"=w684, "Visible"=w683) -> ()  [unwired: 2 in, 2 out]
        n124 = property on="acc" class="Bool (严格)"("Value"=w681, "Visible"=w682) -> ()  [unwired: 2 in, 2 out]
        n125 = property on="ign" class="Bool (严格)"("Value"=w677, "Visible"=w680) -> ()  [unwired: 2 in, 2 out]
        n126 = property on="start" class="Bool (严格)"("Value"=w678, "Visible"=w679) -> ()  [unwired: 2 in, 2 out]
      }
      event Exec State Change {
        n127 = event-data() -> ()  [unwired: 1 in, 4 out]
        n128 = Unbundle By Name(w774) -> ("Run Mode?"=w768:bool)
        n129 = Select(t=u8 1 ("Disabled"), s=w768, f=u8 0 ("Disabled")) -> (s? t:f=w767:u8)
        n130 = property on="SLEEP" class="Bool (严格)"("Disabled"=w767) -> ()  [unwired: 2 in, 2 out]
        n131 = property on="B+" class="Bool (严格)"("Disabled"=w767) -> ()  [unwired: 2 in, 2 out]
        n132 = property on="ACC" class="Bool (严格)"("Disabled"=w767) -> ()  [unwired: 2 in, 2 out]
        n133 = property on="IGN1" class="Bool (严格)"("Disabled"=w767) -> ()  [unwired: 2 in, 2 out]
        n134 = property on="IGN2" class="Bool (严格)"("Disabled"=w767) -> ()  [unwired: 2 in, 2 out]
        n135 = property on="START" class="Bool (严格)"("Disabled"=w767) -> ()  [unwired: 2 in, 2 out]
        n136 = property on="IDLE" class="Bool (严格)"("Disabled"=w767) -> ()  [unwired: 2 in, 2 out]
      }
    }
  }
  "Display State Out" <- w4
  "Data Out" <- w7
  "Action" <- w2
